vi "TeleOp Hanger.vi"() -> ()   [LabVIEW 2020]
uses:
  <vilib>/Rock Robotics/WPI/Utilities/WPI_GetSetVariantRefNum.vi
panel:
  in  "servo rotation":dbl=90.0 format="%#_13g"
  in  "down hanger motor":dbl=-0.5
  in  "up hanger motor":dbl=0.5
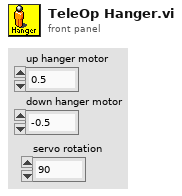
[diagram p1: front panel]
types:
  T1 = typedef "WPI_JoystickDevRef.ctl" = cluster{"Device":T2}
  T2 = typedef "WPI_JoystickDeviceEnum.ctl" = enum16{"USB 0", "USB 1", "USB 2", "USB 3", "USB 4", "USB 5"}
  T3 = typedef "WPI_MotorControlDeviceRef.ctl" = cluster{"DeviceStatus":errorcluster, "Type":T4, "PWM":cluster{"PWM Channel":T5, "DeadBand":T6}, "CAN":cluster{"Device Number":u8, "SetOutput VI Ref":variant, "GetOutput VI Ref":variant, "Enable VI Ref":variant, "Disable VI Ref":variant, "Data":variant}, "Invert":bool, "DIO PWM":cluster{"PWM \"Enable\" Channel":T5, "DIOChannel":T7, "PWM Rate":dbl}}
  T4 = typedef "WPI_MotorControlType.ctl" = enum16{"PWM", "CAN", "DIO PWM"}
  T5 = typedef "FPGA_DIOPWMChannel.ctl" = enum8{"PWM 0", "PWM 1", "PWM 2", "PWM 3", "PWM 4", "PWM 5", "PWM 6", "PWM 7", "PWM 8", "PWM 9", "PWM MXP 0", "PWM MXP 1", "PWM MXP 2", "PWM MXP 3", "PWM MXP 4", "PWM MXP 5", "PWM MXP 6", "PWM MXP 7", "PWM MXP 8", "PWM MXP 9", "Invalid"}
  T6 = typedef "WPI_PWMDeadband.ctl" = cluster{"Name":string, "maxPositivePwm":i32, "minPositivePwm":i32, "centerPwm":i32, "maxNegativePwm":i32, "minNegativePwm":i32, "angularRange":u16}
  T7 = typedef "FPGA_DIOChannel.ctl" = enum8{"DIO 0", "DIO 1", "DIO 2", "DIO 3", "DIO 4", "DIO 5", "DIO 6", "DIO 7", "DIO 8", "DIO 9", "DIO MXP 0", "DIO MXP 1", "DIO MXP 2", "DIO MXP 3", "DIO MXP 4", "DIO MXP 5", "DIO MXP 6", "DIO MXP 7", "DIO MXP 8", "DIO MXP 9", "DIO MXP 10", "DIO MXP 11", "DIO MXP 12", "DIO MXP 13", "DIO MXP 14", "DIO MXP 15", "SPI Port CS1", "SPI Port CS2", "SPI Port CS3", "SPI Port MISO", "SPI Port MOSI", "Invalid"}
  T8 = typedef "WPI_ServoDeviceRef.ctl" = cluster{"DeviceStatus":errorcluster, "PWM Channel":T5, "DeadBand":T6}
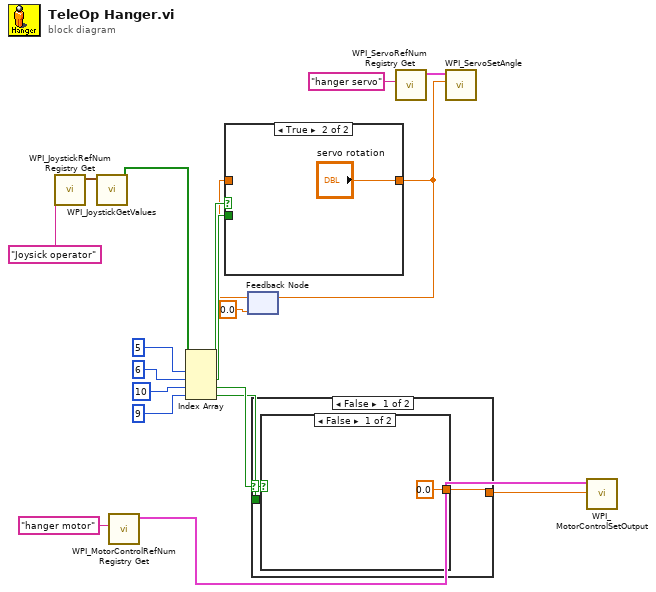
[diagram p0: block diagram]
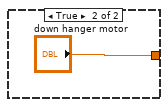
[diagram p2: hidden frame]
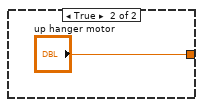
[diagram p3: hidden frame]
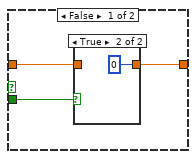
[diagram p4: hidden frame]
diagram:
  n1 = call <vilib>:"WPI_JoystickRefNum Registry Get.vi"("refnum name"="Joysick operator") -> ("JoystickDevRef"=w16:T1)  [unwired: 9 in, 1 out]
  n2 = call <vilib>:"WPI_JoystickGetValues.vi"("JoystickDevRef"=w16) -> ("Buttons"=w17:bool[])  [unwired: 6 in, 4 out]
  n3 = call <vilib>:"WPI_MotorControlRefNum Registry Get.vi"("refnum name"="hanger motor") -> ("MotorControlDevRef"=w2:T3)  [unwired: 9 in, 1 out]
  n4 = Index Array(array=w17, index #1=5 ("index"), index #2=6 ("index"), index #3=10 ("index"), index #4=9 ("index")) -> (element #1=w11:bool, element #2=w10:bool, element #3=w5:bool, element #4=w4:bool)
  n5 = feedback #1(0.0) -> (w7:dbl)
  n6 = case shown="True" w11 {
    tunnel: w10 -> [w22 _]
    tunnel: [w21 "servo rotation"] -> w8
    tunnel: w7 -> [w20 _]
    frame False {
      n7 = case shown="True" w22 {
        tunnel: [w23 0] -> w21
        tunnel: w20 -> [w23 _]
        frame False {
        }
        frame True {
        }
      }
    }
    frame True {
    }
  }
  n8 = feedback-in #1(w8) -> ()
  n9 = case shown="False" w5 {
    tunnel: w4 -> [w27 _]
    tunnel: [w26 "up hanger motor"] -> w1
    frame False {
      n10 = case shown="False" w27 {
        tunnel: [0.0 ("down hanger motor") "down hanger motor"] -> w26
        frame False {
        }
        frame True {
        }
      }
    }
    frame True {
    }
  }
  n11 = call <vilib>:"WPI_ServoRefNum Registry Get.vi"("refnum name"="hanger servo") -> ("ServoDeviceRef"=w9:T8)  [unwired: 9 in, 1 out]
  n12 = call <vilib>:"WPI_ServoSetAngle.vi"("Angle"=w8, "ServoDeviceRef"=w9) -> ()  [unwired: 8 in, 2 out]
  n13 = call <vilib>:"WPI_MotorControlSetOutput.vi"("Output"=w1, "MotorControlDevRef"=w2) -> ()  [unwired: 7 in, 3 out]
